vi "Do This.vi"(8 "error in (no error)":errorcluster, 10 "Status Events":refnum<class "Status Events.lvclass">, 11 "VIP Uninstall in":refnum<class "VIP Uninstall.lvclass">) -> (0 "error out":errorcluster, 3 "VIP Uninstall out":refnum<class "VIP Uninstall.lvclass">)   [LabVIEW 2014, in "VIP Uninstall.lvclass"]
uses:
  VIP Uninstall.lvclass
  Shared/Classes/Status Events/Status Events.lvclass
  VIP Uninstall.lvclass/VIP Uninstall.ctl
  <vilib>/Utility/error.llb/DialogType.ctl
  Classes/Job/Job.lvclass/Job.ctl
  <vilib>/JKI/VIPM API/VIPM API_vipm_api.lvlib
  Classes/Job/Job.lvclass
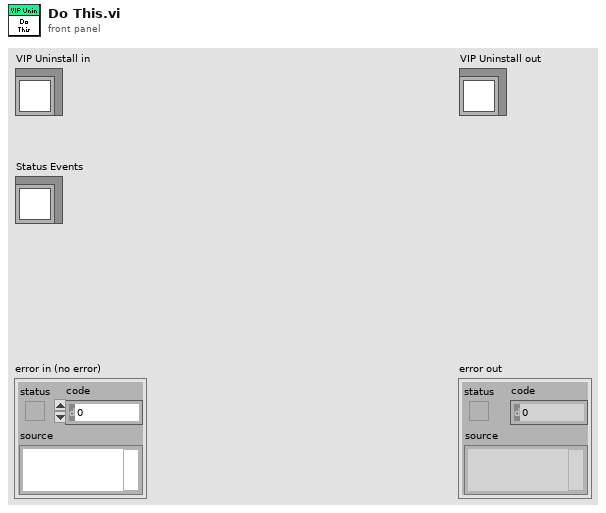
[diagram p1: front panel]
types:
  T1 = typedef "VIPM API_vipm_api.lvlib/Library Contents Cluster_vipm_api.ctl" = cluster{"Package Name":string, "Version":string, "Display Name":string, "Repository Name":string, "Company Name":string, "License Type":string, "Installed":bool, "Deprecated":bool, "Dependency or Conflict Problem":bool, "Downloaded":bool}
  T2 = typedef "DialogType.ctl" = u16
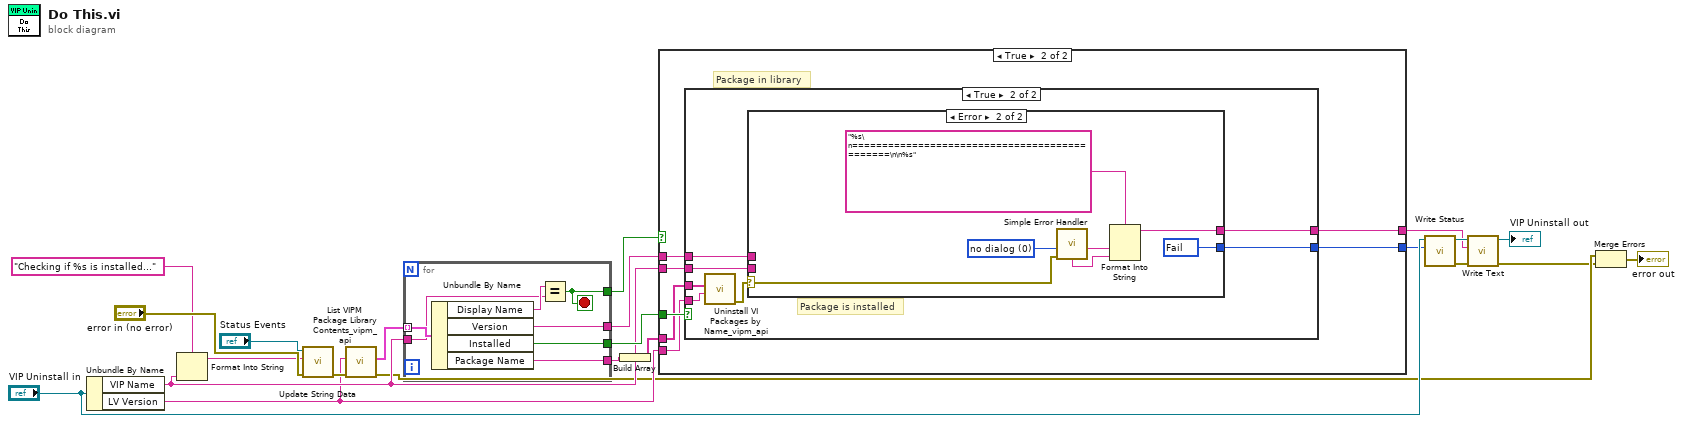
[diagram p0: block diagram]
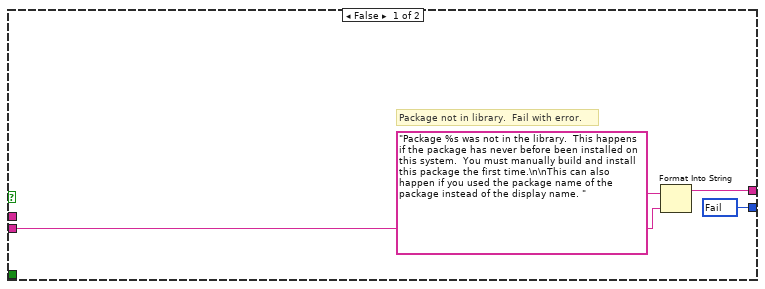
[diagram p2: hidden frame]
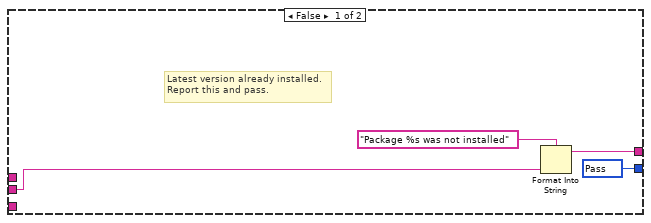
[diagram p3: hidden frame]
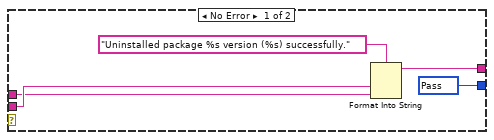
[diagram p4: hidden frame]
diagram:
  n1 = Unbundle By Name("VIP Uninstall in") -> ("VIP Name"=w10:string, "LV Version"=w7:string)
  n2 = Format Into String(format string="Checking if %s is installed...", w10) -> (resulting string=w19:string)  [unwired: 2 in, 1 out]
  n3 = call "Update String Data.vi"("error in (no error)"="error in (no error)", "String Data"=w19, "Status Updater in"="Status Events") -> ("error out"=w18:errorcluster)  [unwired: 7 in, 1 out]
  n4 = call <vilib>:"List VIPM Package Library Contents_vipm_api.vi"("error in (no error)"=w18, "LabVIEW Version"=w7) -> ("error out"=w4:errorcluster, "Library Contents []"=w17:T1[])  [unwired: 8 in]
  n5 = for {
    tunnel: w17 -> [w29] mode=indexing
    tunnel: w10 -> [w27]
    tunnel: [w26] -> w15
    tunnel: [w24] -> w9
    tunnel: [w25] -> w16
    tunnel: [w23] -> w1
    stop <- w25 stop-if-true
    n6 = Unbundle By Name(w29) -> ("Display Name"=w28:string, "Version"=w24:string, "Installed"=w26:bool, "Package Name"=w23:string)
    n7 = Equal?(x=w28, y=w27) -> (x = y?=w25:bool)
  }
  n8 = Build Array(w1) -> (w8:string[])
  n9 = case shown="True" w16 {
    tunnel: w15 -> [_ w40]
    tunnel: w10 -> [w30 w39]
    tunnel: w9 -> [_ w38]
    tunnel: [w33 w37] -> w6
    tunnel: w8 -> [_ w36]
    tunnel: w7 -> [_ w35]
    tunnel: [w31 w34] -> w5
    frame False {
      w33 = u16 500 items=["Abort"=503, "Fail"=500, "Pass"=200] ("Status")
      # "Package not in library.  Fail with error."
      n10 = Format Into String(format string="Package %s was not in the library.  This happens if the package has never before been installed on this system.  You must manually build and install this package the first time.\n\nThis can also happen if you used the package name of the package instead of the display name. ", w30) -> (resulting string=w31:string)  [unwired: 2 in, 1 out]
    }
    frame True {
      # "Package in library"
      n11 = case shown="True" w40 {
        tunnel: w39 -> [w41 w46]
        tunnel: w38 -> [_ w45]
        tunnel: [w43 w48] -> w37
        tunnel: w36 -> [_ w51]
        tunnel: w35 -> [_ w50]
        tunnel: [w42 w47] -> w34
        frame False {
          w43 = u16 200 items=["Abort"=503, "Fail"=500, "Pass"=200] ("Status")
          # "Latest version already installed.\nReport this and pass."
          n12 = Format Into String(format string="Package %s was not installed", w41) -> (resulting string=w42:string)  [unwired: 2 in, 1 out]
        }
        frame True {
          # "Package is installed"
          n13 = call <vilib>:"Uninstall VI Packages by Name_vipm_api.vi"("LabVIEW Version"=w50, "Package Names to Uninstall []"=w51) -> ("error out"=w49:errorcluster)  [unwired: 9 in]
          n14 = case shown="Error" w49 {
            selector: w49 -> [_ w57]
            tunnel: [w56 w63] -> w48
            tunnel: [w54 w58] -> w47
            tunnel: w46 -> [w53 _]
            tunnel: w45 -> [w52 _]
            frame No Error {
              w56 = u16 200 items=["Abort"=503, "Fail"=500, "Pass"=200] ("Status")
              n15 = Format Into String(format string="Uninstalled package %s version (%s) successfully.", w53, w52) -> (resulting string=w54:string)  [unwired: 2 in, 1 out]
            }
            frame Error {
              w59 = T2 0 items=["no dialog", "OK message", "continue or stop message", "OK message + warnings", "continue/stop + warnings"] ("type of dialog (OK msg:1)")
              w63 = u16 500 items=["Abort"=503, "Fail"=500, "Pass"=200] ("Status")
              n16 = call <vilib>:"Simple Error Handler.vi"("type of dialog (OK msg:1)"=w59, "error in (no error)"=w57) -> ("source out"=w61:string, "message"=w62:string)  [unwired: 3 in, 3 out]
              n17 = Format Into String(format string="%s\n==============================================\n\n%s", w61, w62) -> (resulting string=w58:string)  [unwired: 2 in, 1 out]
            }
          }
        }
      }
    }
  }
  n18 = call "Write Status.vi"("Status"=w6, "Job in"="VIP Uninstall in") -> ("error out"=w12:errorcluster, "Job out"=w13:refnum<class "VIP Uninstall.lvclass">)  [unwired: 8 in]
  n19 = call "Write Text.vi"("error in (no error)"=w12, "Text"=w5, "Job in"=w13) -> ("error out"=w3:errorcluster, "Job out"=→"VIP Uninstall out":refnum<class "VIP Uninstall.lvclass">)  [unwired: 7 in]
  n20 = Merge Errors(w4, w3) -> (→"error out":errorcluster)
